vi "ProtectBall.vi"(8 "error in (no error)":errorcluster, 11 "Protect Ball in":refnum<class "Protect Ball.lvclass">) -> (0 "error out":errorcluster, 3 "Protect Ball out":refnum<class "Protect Ball.lvclass">)   [LabVIEW 2022 SP3, in "Protect Ball.lvclass"]
uses:
  Protect Ball.lvclass
  C:/Users/ebert/Documents/codes/SSL/repo/SSL_AI/GoToSkill_class/GoToSkill.lvclass
  Robot_class/Robot.lvclass
  Game_class/Game.lvclass
  Game_class/Game.lvclass/Game.ctl
  Team_class/Team.lvclass/Team.ctl
  Game_class/Read BallRef.vi
  Game_class/Read EnemyRef.vi
  Team_class/Read RobotRef.vi
  Enemy_class/Enemy.lvclass
  C:/Users/ebert/Documents/codes/SSL/repo/SSL_AI/Team_class/Team.lvclass
  Ball_class/Ball.lvclass
  GoToSkill_class/GoToSkill.lvclass
  Utilities_class/Utilities.lvclass
panel:
  in  "Game":refnum<class "Game.lvclass">
  in  "Robot in":refnum<class "Robot.lvclass">
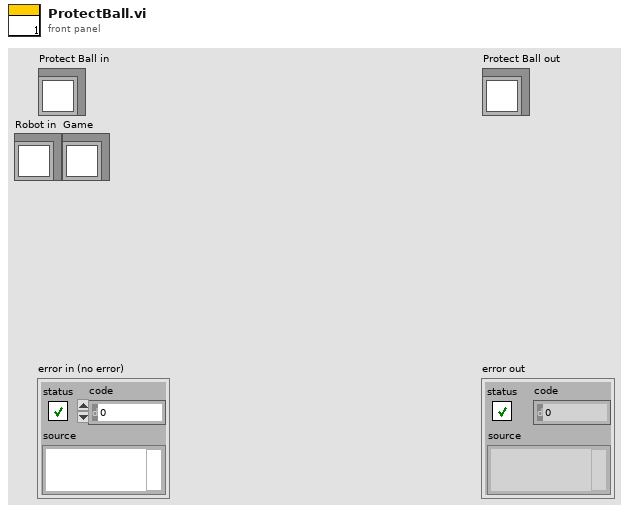
[diagram p1: front panel]
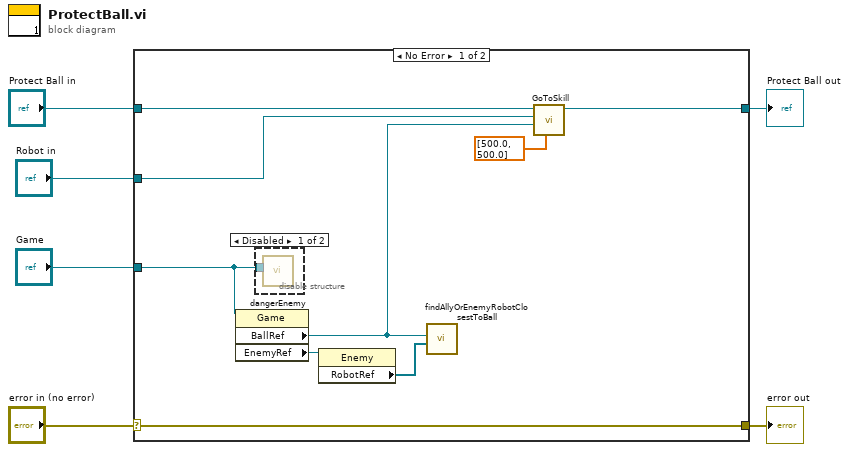
[diagram p0: block diagram]
diagram:
  n1 = case shown="No Error" "error in (no error)" {
    selector: "error in (no error)" -> [w15 w18]
    tunnel: [w15 w18] -> w5
    tunnel: [w12 w17] -> w3
    tunnel: "Protect Ball in" -> [w14 w17]
    tunnel: "Robot in" -> [w13 _]
    tunnel: "Game" -> [w11 _]
    frame No Error {
      n2 = property class="Game"(reference=w11) -> ("BallRef"=w8:refnum<class "Ball.lvclass">, "EnemyRef"=w10:refnum<class "Enemy.lvclass">)  [unwired: 1 in, 2 out]
      n3 = disable-structure shown="Disabled" {
        disable-tunnel: w11 -> [w16 _]
        frame Disabled {
          n4 = call "dangerEnemy.vi"("Game"=w16) -> ()  [unwired: 4 in, 7 out]
        }
        frame Enabled {
        }
      }
      n5 = property class="Enemy"(reference=w10) -> ("RobotRef"=w9:refnum<class "Robot.lvclass">[])  [unwired: 1 in, 2 out]
      n6 = call "findAllyOrEnemyRobotClosestToBall.vi"("Ally/Enemy Robots"=w9, "Ball"=w8) -> ()  [unwired: 6 in, 4 out]
      n7 = call "GoToSkill.vi"("Position"=dbl[] [500.0, 500.0], "BallRef"=w8, "Robot in"=w13, "GoToSkill in"=w14) -> ("GoToSkill out"=w12:refnum<class "Protect Ball.lvclass">)  [unwired: 5 in, 2 out]
    }
    frame Error {
    }
  }
  "error out" <- w5
  "Protect Ball out" <- w3
